vi "dfd_Error Cluster From Error Code (Array).vi"(8 "error in (no error)":errorcluster, 11 "error code (0)":i32[](array[numeric])) -> (0 "error out":errorcluster)   [LabVIEW 2017, in "NI_DigFilterLicensed.lvlib"]
uses:
  <vilib>/addons/Digital Filter Design/NI_DigFilterLicensed.lvlib
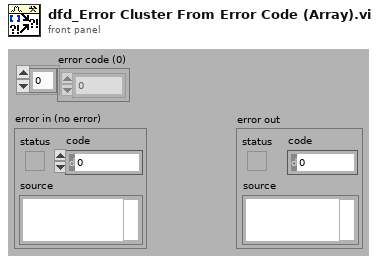
[diagram p1: front panel]
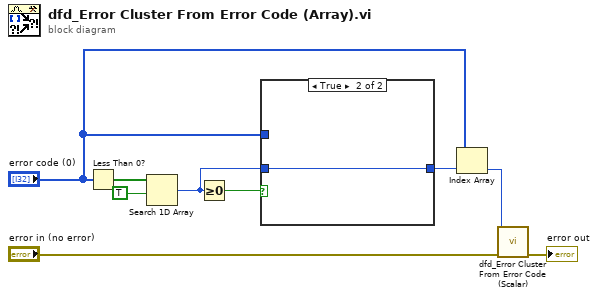
[diagram p0: block diagram]
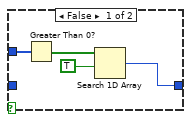
[diagram p2: hidden frame]
diagram:
  n1 = Less Than 0?(x="error code (0)") -> (x < 0?=w9:bool[])
  n2 = Search 1D Array(1D array=w9, element=TRUE) -> (index of element=w3:i32)  [unwired: 1 out]
  n3 = Greater Or Equal To 0?(x=w3) -> (x >= 0?=w5:bool)
  n4 = case shown="True" w5 {
    tunnel: "error code (0)" -> [w13 _]
    tunnel: [w10 w14] -> w4
    tunnel: w3 -> [_ w14]
    frame False {
      n5 = Greater Than 0?(x=w13) -> (x > 0?=w11:bool[])
      n6 = Search 1D Array(1D array=w11, element=TRUE) -> (index of element=w10:i32)  [unwired: 1 out]
    }
    frame True {
    }
  }
  n7 = Index Array(array="error code (0)", index=w4) -> (element=w1:i32)
  n8 = call <vilib>:"dfd_Error Cluster From Error Code (Scalar).vi"("error in (no error)"="error in (no error)", "error code (0)"=w1) -> ("error out"=→"error out":errorcluster)  [unwired: 9 out]
